vi "demo.vi"() -> ()   [LabVIEW 2010]
uses:
  password.xctl
panel:
  in  "password":string(xcontrol)
  out "password value":string
  in  "delay":u32=2000
  # "delay after witch a newly typed\ncharacter will be replaced with a star"
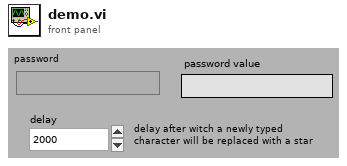
[diagram p1: front panel]
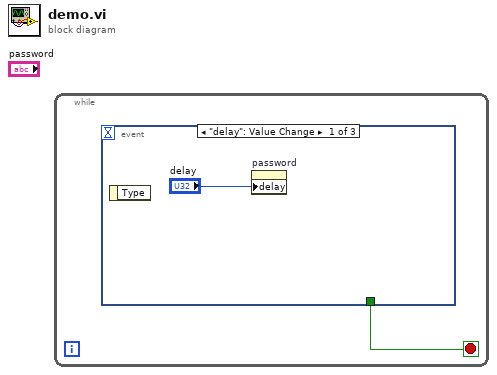
[diagram p0: block diagram]
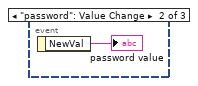
[diagram p2: hidden frame]
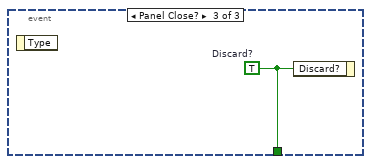
[diagram p3: hidden frame]
diagram:
  n1 = while {
    stop <- w1 stop-if-true
    n2 = event shown="[0] \"delay\": Value Change" {
      selector: _ -> [_ _ _]
      dyn-events: _ -> [_ _ _]
      timeout: _ -> [_ _ _]
      tunnel: [_ _ w4] -> w1
      event "delay": Value Change {
        n3 = event-data() -> ()  [unwired: 1 in, 1 out]
        n4 = property on="password" class="password (strict)"("delay"="delay") -> ()  [unwired: 2 in, 2 out]
      }
      event "password": Value Change {
        n5 = event-data() -> ("NewVal"=→"password value":string)  [unwired: 1 in]
      }
      event Panel Close? {
        w4 = TRUE  # Discard?
        n6 = event-data() -> ()  [unwired: 1 in, 1 out]
        n7 = event-data("Discard?"=w4) -> ()  [unwired: 1 in, 1 out]
      }
    }
  }
